vi "e.gate Decode UDBF - Stream.vi"(8 "error in (no error)":errorcluster, 10 "DecodeTimeFormat":string, 11 "UDBF Stream":string) -> (0 "error out":errorcluster, 2 "data array (double)":dbl[][](array[numeric]), 3 "Configuration out":T1 {"StartTime" format="%#.10f"; "dActTimeToSecondFactor" format="%#.10f"; "StartTimeToDayFactor" format="%#_10f"})   [LabVIEW 2016]
doc: "This VI is used to decode a UDBF data stream with header and data merged together."
uses:
  e.gate Configuration.ctl
  e.gate Channel Data.ctl
  e.gate Data Type.ctl
  e.gate Protocol Type.ctl
  e.gate Module  Data.ctl
  e.gateHSP_DLLhandle.ctl
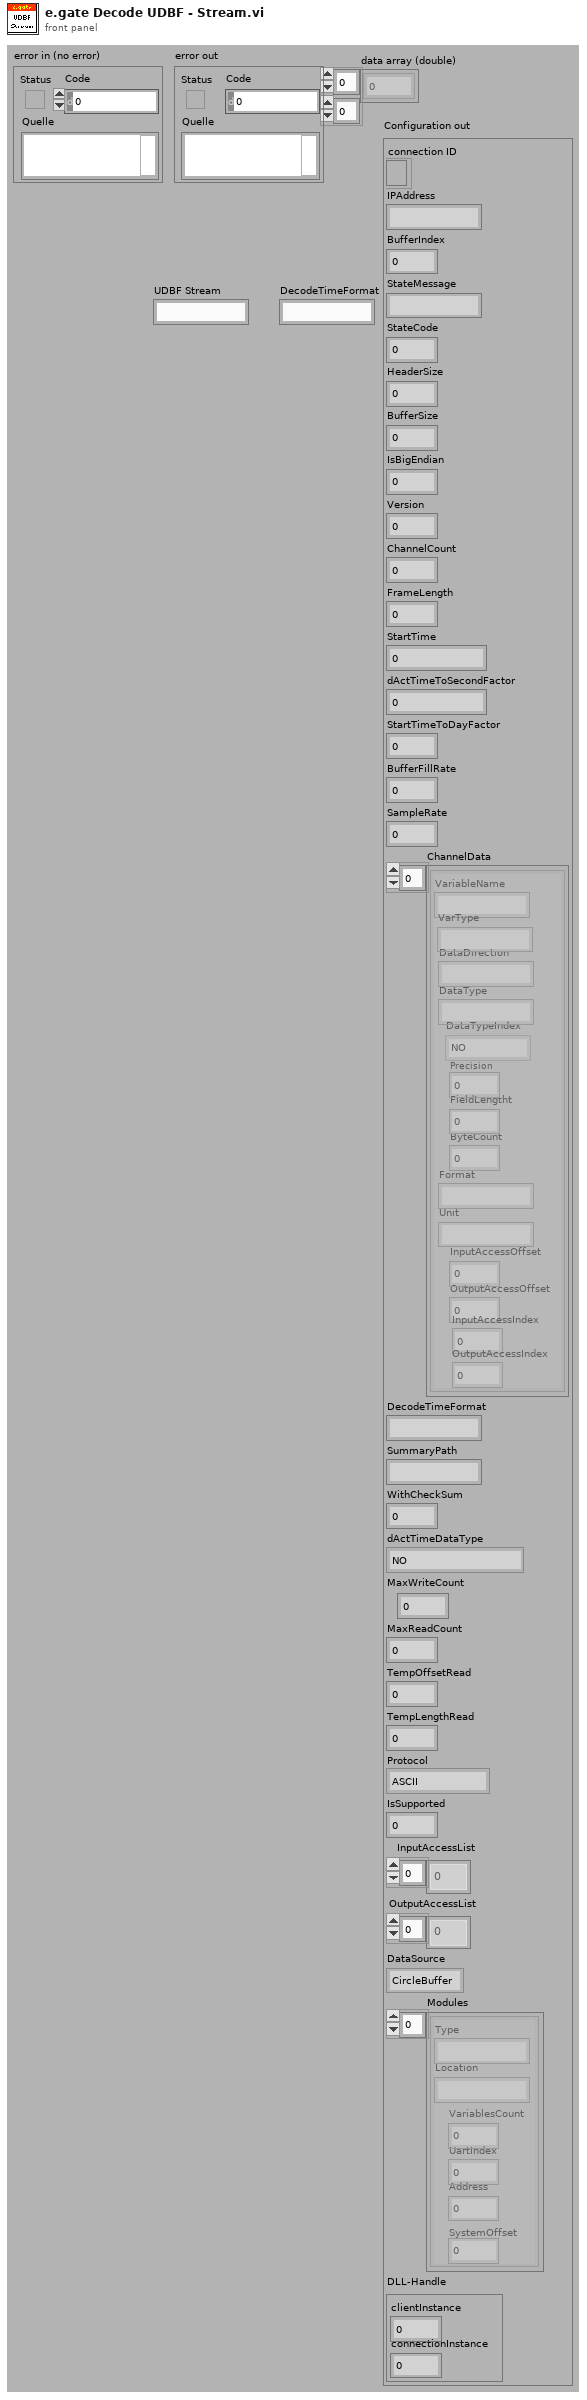
[diagram p1: front panel]
types:
  T1 = typedef "e.gate Configuration.ctl" = cluster{"connection ID":refnum<k5>, "IPAddress":string, "BufferIndex":i32, "StateMessage":string, "StateCode":i8, "HeaderSize":i32, "BufferSize":i32, "IsBigEndian":i32, "Version":i32, "ChannelCount":i32, "FrameLength":i32, "StartTime":dbl, "dActTimeToSecondFactor":dbl, "StartTimeToDayFactor":dbl, "BufferFillRate":dbl, "SampleRate":dbl, "ChannelData":T2[], "DecodeTimeFormat":string, "SummaryPath":string, "WithCheckSum":i32, "dActTimeDataType":T3, "MaxWriteCount":i32, "MaxReadCount":i32, "TempOffsetRead":i32, "TempLengthRead":i32, "Protocol":T4, "IsSupported":i32, "InputAccessList":i32[], "OutputAccessList":i32[], "DataSource":enum16{"CircleBuffer", "test.con Logger", "test.con Archive"}, "Modules":T5[], "DLL-Handle":T6}
  T2 = typedef "e.gate Channel Data.ctl" = cluster{"VariableName":string, "DataDirection":string, "DataType":string, "DataTypeIndex":T3, "Precision":i16, "FieldLengtht":i16, "ByteCount":i32, "Format":string, "Unit":string, "InputAccessOffset":i32, "OutputAccessOffset":i16, "InputAccessIndex":i16, "OutputAccessIndex":i16, "VarType":string}
  T3 = typedef "e.gate Data Type.ctl" = enum16{"NO", "BOOL", "SINT8", "USINT8", "SINT16", "USINT16", "SINT32", "USINT32", "FLOAT", "SET8", "SET16", "SET32", "DOUBLE", "SINT64", "USINT64", "SET64"}
  T4 = typedef "e.gate Protocol Type.ctl" = enum16{"ASCII", "HighspeedPort Online", "HighspeedPort Buffer", "eGateHighspeedPortDLL "}
  T5 = typedef "e.gate Module  Data.ctl" = cluster{"Type":string, "Location":string, "VariablesCount":i16, "UartIndex":i16, "Address":i16, "SystemOffset":i16}
  T6 = typedef "e.gateHSP_DLLhandle.ctl" = cluster{"clientInstance":i32, "connectionInstance":i32}
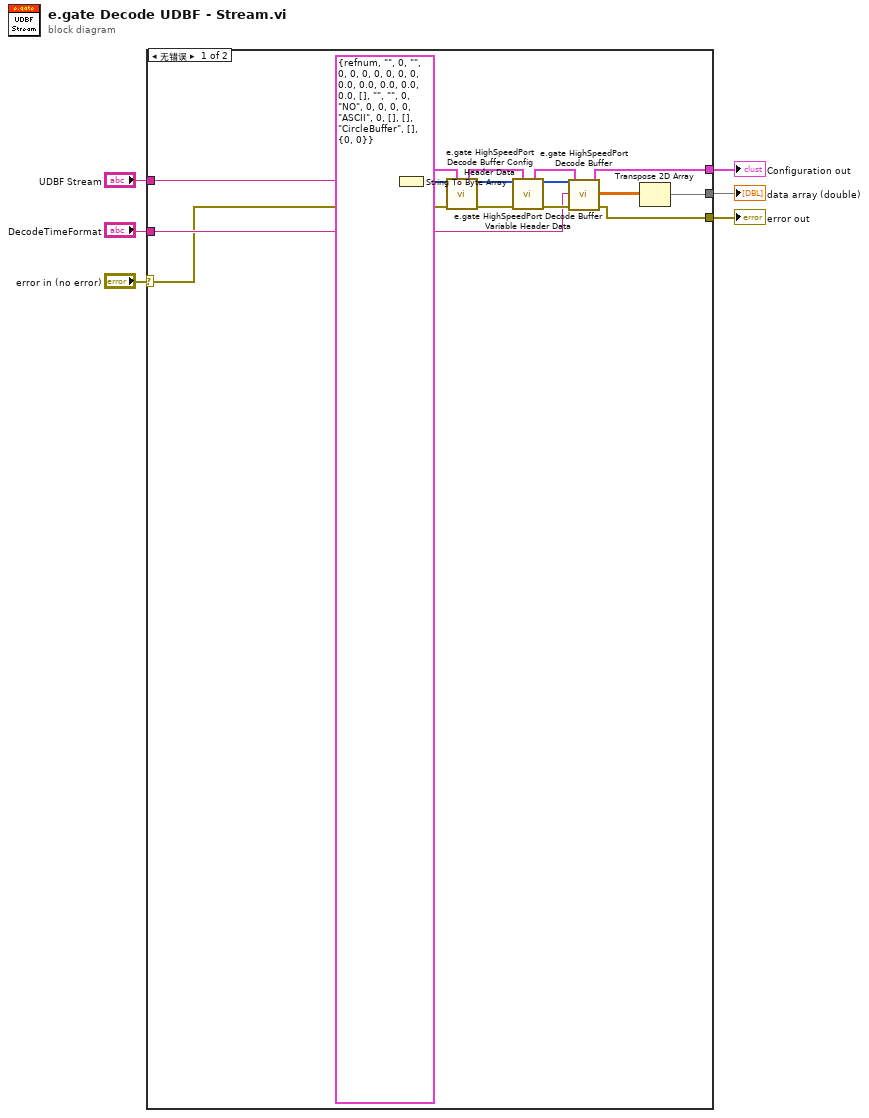
[diagram p0: block diagram]
diagram:
  n1 = case shown="无错误" "error in (no error)" {
    selector: "error in (no error)" -> [w11 w22]
    tunnel: "DecodeTimeFormat" -> [w14 _]
    tunnel: "UDBF Stream" -> [w13 _]
    tunnel: [w8 _] -> w3
    tunnel: [w10 _] -> w2
    tunnel: [w9 w22] -> w1
    frame No Error {
      n2 = String To Byte Array(string=w13) -> (unsigned byte array=w17:u8[])
      n3 = call "e.gate HighSpeedPort Decode Buffer Config Header Data.vi"("Data in (binary)"=w17, "Configuration in"=T1 {"connection ID"=refnum, "IPAddress"="", "BufferIndex"=0, "StateMessage"="", "StateCode"=0, "HeaderSize"=0, "BufferSize"=0, "IsBigEndian"=0, "Version"=0, "ChannelCount"=0, "FrameLength"=0, "StartTime"=0.0, "dActTimeToSecondFactor"=0.0, "StartTimeToDayFactor"=0.0, "BufferFillRate"=0.0, "SampleRate"=0.0, "ChannelData"=[], "DecodeTimeFormat"="", "SummaryPath"="", "WithCheckSum"=0, "dActTimeDataType"=enum."NO", "MaxWriteCount"=0, "MaxReadCount"=0, "TempOffsetRead"=0, "TempLengthRead"=0, "Protocol"=enum."ASCII", "IsSupported"=0, "InputAccessList"=[], "OutputAccessList"=[], "DataSource"=enum."CircleBuffer", "Modules"=[], "DLL-Handle"={"clientInstance"=0, "connectionInstance"=0}} ("e.gate Configuration"), "error in (no error)"=w11) -> ("Configuration out"=w19:T1, "Data out (binary)"=w21:u8[], "error out"=w20:errorcluster)  [unwired: 10 out]
      n4 = call "e.gate HighSpeedPort Decode Buffer Variable Header Data.vi"("Data in (binary)"=w21, "Configuration in"=w19, "error in (no error)"=w20) -> ("Configuration out"=w16:T1, "Remaining Data out"=w12:u8[], "error out"=w15:errorcluster)  [unwired: 10 out]
      n5 = call "e.gate HighSpeedPort Decode Buffer.vi"("Data in (binary)"=w12, "DecodeTimeFormat"=w14, "error in"=w15, "Configuration  in"=w16) -> ("Configuration out"=w10:T1, "data array (double)"=w7:dbl[][], "error out"=w9:errorcluster)  [unwired: 21 out]
      n6 = Transpose 2D Array(2D array=w7) -> (transposed array=w8:dbl[][])
    }
    frame Error {
    }
  }
  "data array (double)" <- w3
  "Configuration out" <- w2
  "error out" <- w1
